vi "给表格单元格上色.vi"(8 "错误输入（无错误）":errorcluster, 9 "选中颜色盒":u32(colorbox)=12439011, 10 "坐标":T1={"Row"=20, "Column"=20} caption="本次坐标", 11 "引用输入":refnum<vi>) -> (0 "错误输出":errorcluster, 3 "引用输出":refnum<vi>)   [LabVIEW 2014, in "表格.lvlib" / "表格上色.lvlib"]
uses:
  <vilib>/Utility/miscctls.llb/LVRowAndColumnTypeDef.ctl
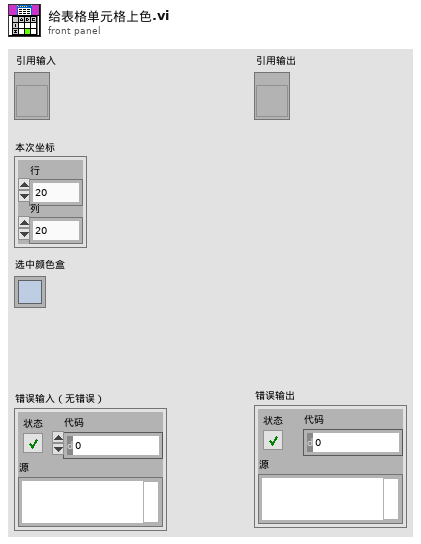
[diagram p1: front panel]
types:
  T1 = typedef "LVRowAndColumnTypeDef.ctl" = cluster{"Row":i32, "Column":i32}
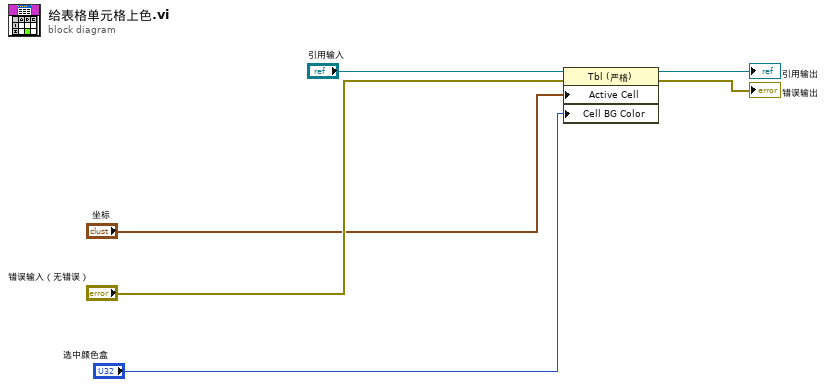
[diagram p0: block diagram]
diagram:
  n1 = property on="属性节点" class="Tbl (严格)"(reference="引用输入", error in="错误输入（无错误）", "Active Cell"="坐标", "Cell BG Color"="选中颜色盒") -> (reference out=→"引用输出":refnum<vi>, error out=→"错误输出":errorcluster)
